vi "List Blobs.vi"(8 "error in (no error)":errorcluster, 10 "Container":string, 11 "Azure Session in":refnum<class "Session.lvclass">) -> (0 "error out":errorcluster, 2 "Blobs":string[](array[string]), 3 "Azure Session out":refnum<class "Session.lvclass">)   [LabVIEW 2015, in "NI_Azure_Blob.lvlib"]
doc: "Lists all of the blobs in a container."
uses:
  NI_Azure_Blob.lvlib
  Core/Session/Session.lvclass
  Core/Name Value Pair.ctl
  Core/Session/Session.lvclass/Session.ctl
  Core/Session/Write Request Parameters.vi
  Core/Session/Write HTTP Verb.vi
  Core/Session/Write URL Suffix.vi
  Core/NI_Azure_Core.lvlib
  XML Parsing/NI_Azure_XML Parsing.lvlib
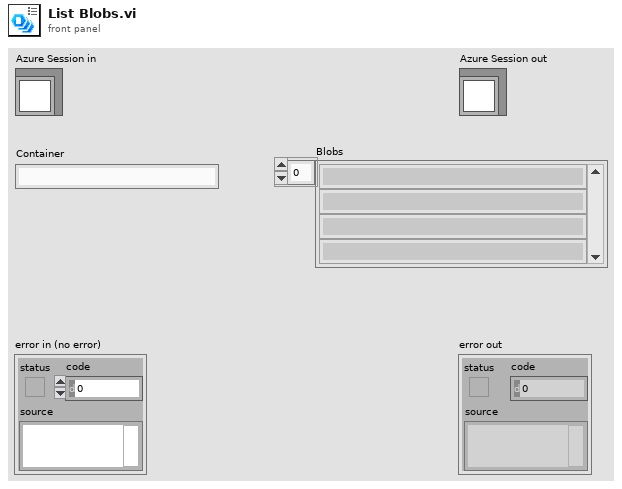
[diagram p1: front panel]
types:
  T1 = typedef "NI_Azure_Core.lvlib/Name Value Pair.ctl" = cluster{"name":string, "value":string}
  T2 = typedef "NI_Azure_Core.lvlib/Response.ctl" = cluster{"Headers":string, "Body":string}
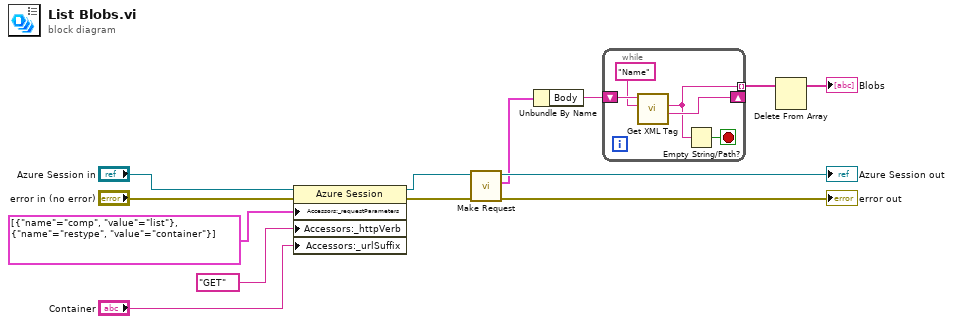
[diagram p0: block diagram]
diagram:
  n1 = property class="Azure Session"(reference="Azure Session in", error in="error in (no error)", "Accessors:_requestParameters"=T1[] [{"name"="comp", "value"="list"}, {"name"="restype", "value"="container"}] ("request parameters"), "Accessors:_httpVerb"="GET" ("HTTP-Verb"), "Accessors:_urlSuffix"="Container") -> (reference out=w4:refnum<class "Session.lvclass">, error out=w6:errorcluster)
  n2 = call "Make Request.vi"("error in (no error)"=w6, "Session in"=w4) -> ("error out"=→"error out":errorcluster, "Response"=w7:T2, "Session out"=→"Azure Session out":refnum<class "Session.lvclass">)  [unwired: 7 in]
  n3 = Unbundle By Name(w7) -> ("Body"=w8:string)
  n4 = while {
    shift-right: [w17] -> _
    shift-left: w8 -> [w18]
    tunnel: [w15] -> w9 mode=indexing
    stop <- w14 stop-if-true
    n5 = call "Get XML Tag.vi"("Tag name"="Name", "XML String in"=w18) -> ("Remaining string"=w17:string, "Tag value"=w15:string)  [unwired: 5 in, 3 out]
    n6 = Empty String/Path?(string/path=w15) -> (empty?=w14:bool)
  }
  n7 = Delete From Array(array=w9) -> (array with subset deleted=→"Blobs":string[])  [unwired: 2 in, 1 out]
